vi "In Place Read String.vi"(8 "error in (no error)":errorcluster, 9 "offset (0)":i64, 10 "preallocated string in":string, 11 "pointer in":u64) -> (0 "error out":errorcluster, 1 "offset out":i64, 2 "string out":string, 3 "pointer out":u64)   [LabVIEW 2016, in "Linux RT IPC.Shared Memory.lvlib"]
uses:
  Linux RT IPC.Shared Memory.lvlib
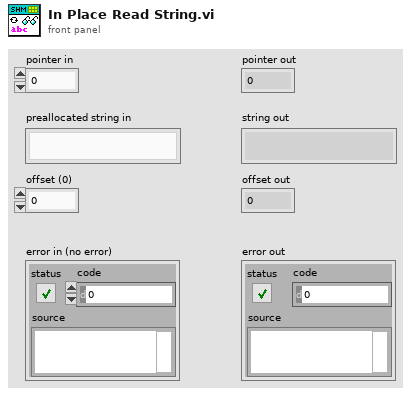
[diagram p1: front panel]
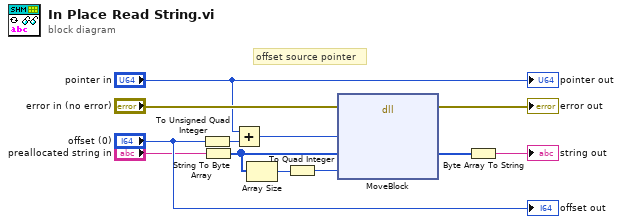
[diagram p0: block diagram]
diagram:
  # "offset source pointer"
  n1 = To Unsigned Quad Integer(1:"offset (0)") -> (0:w8:u64)
  n2 = String To Byte Array(string="preallocated string in") -> (unsigned byte array=w3:u8[])
  n3 = Add(x="pointer in", y=w8) -> (x+y=w7:u64)
  n4 = Array Size(array=w3) -> (size(s)=w2:i32)
  n5 = To Quad Integer(1:w2) -> (0:w1:i64)
  n6 = dll-call lib="LabVIEW" fn="MoveBlock"(error in="error in (no error)", "pointer"=w7, "data"=w3, "size"=w1) -> (error out=→"error out":errorcluster, "data"=w6:u8[])  [unwired: 5 in, 1 out]
  n7 = Byte Array To String(unsigned byte array=w6) -> (string=→"string out":string)
  "pointer out" <- "pointer in"
  "offset out" <- "offset (0)"
